vi "MissingIndicator.vi"(8 "error in":errorcluster caption="entrée d'erreur", 11 "MissingIndicator":T1={"missing_values"="nan", "features"="None", "sparse"="None", "error_on_new"=TRUE}) -> (0 "error out":errorcluster caption="sortie d'erreur", 3 "MissingIndicator.lvclass":refnum<class "MissingIndicator.lvclass">)   [LabVIEW 2020]
doc: "Binary indicators for missing values.\n\nNote that this component typically should not be used in a vanilla Pipeline consisting of transformers and a classifier, but rather could be added using a FeatureUnion or ColumnTransformer.\n\nParameters :\n\n- missing_values : number, string, np.nan (default) or None\nThe placeholder for the missing values. All occurrences of missing_values will be imputed. For pandas’ dataframes with nullable integer dtypes with missing values, missing_values should be set to np.nan, since pd.NA will be converted to np.nan.\n\n- features : str, default=None\nWhether the imputer mask should represent all or a subset of features.\n\nIf “missing-only” (default), the imputer mask will only represent features containing missing values during fit time.\n\nIf “all”, the imputer mask will represent all features.\n\n- sparse : boolean or “auto”, default=None\nWhether the imputer mask format should be sparse or dense.\n\nIf “auto” (default), the imputer mask will be of same type as input.\n\nIf True, the imputer mask will be a sparse matrix.\n\nIf False, the imputer mask will be a numpy array.\n\n- error_on_new : boolean, default=None\nIf True (default), transform will raise an error when there are features with missing values in transform that have no missing values in fit. This is applicable only when features=\"missing-only\".\n\n\n\nMethods : \n\n- Fit : Fit the transformer on X.\n\nParameters : X : {array-like, sparse matrix}, shape (n_samples, n_features)\n Input data, where n_samples is the number of samples and n_features is the number of features.\n\n\n- Fit Transform : Generate missing values indicator for X.\n\nParameters : X : {array-like, sparse matrix}, shape (n_samples, n_features)\n The input data to complete.\n\nReturns : Xt {ndarray or sparse matrix}, shape (n_samples, n_features) or (n_samples, n_features_with_missing)\n The missing indicator for input data. The data type of Xt will be boolean.\n\n\n- Transform : Generate missing values indicator for X.\n\nParameters : X : {array-like, sparse matrix}, shape (n_samples, n_features)\n The input data to complete.\n\nReturns : Xt : {ndarray or sparse matrix}, shape (n_samples, n_features) or (n_samples, n_features_with_missing)\n The missing indicator for input data. The data type of Xt will be boolean."
uses:
  MissingIndicator.lvclass
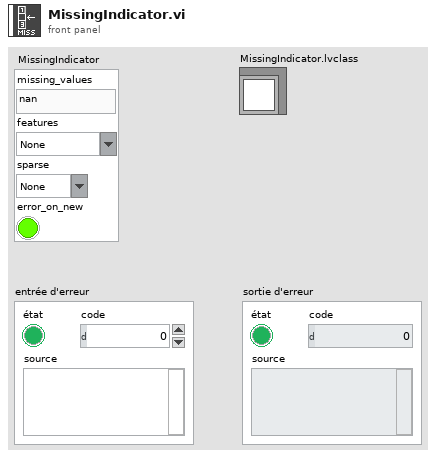
[diagram p1: front panel]
types:
  T1 = cluster{"missing_values":string, "features":string, "sparse":string, "error_on_new":bool}
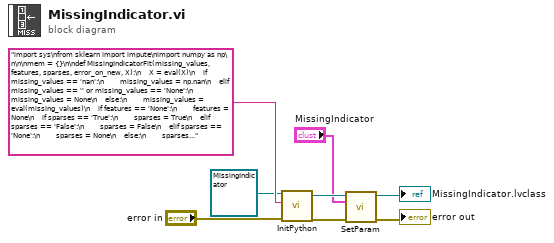
[diagram p0: block diagram]
diagram:
  n1 = call-dynamic "InitPython.vi"("error in (no error)"="error in", "Python Instruction"="import sys\nfrom sklearn import impute\nimport numpy as np\n\n\nmem = {}\n\ndef MissingIndicatorFit(missing_values, features, sparses, error_on_new, X):\n    X = eval(X)\n    if missing_values == 'nan':\n        missing_values = np.nan\n    elif missing_values == '' or missing_values == 'None':\n        missing_values = None\n    else:\n        missing_values = eval(missing_values)\n    if features == 'None':\n        features = None\n    if sparses == 'True':\n        sparses = True\n    elif sparses == 'False':\n        sparses = False\n    elif sparses == 'None':\n        sparses = None\n    else:\n        sparses = 'auto'\n    try:\n        MissingIndicator = impute.MissingIndicator(missing_values, features, sparses, error_on_new).fit(X)\n        mem['FitMissingIndicator'] = MissingIndicator\n        return str('OK')\n    except:\n        erreur = sys.exc_info()\n        typerr = u\"%s\" % (erreur[0])\n        typerr = typerr[typerr.find(\"'\")+1:typerr.rfind(\"'\")]\n        msgerr = u\"%s\" % (erreur[1])\n        message = str('/!\\\\ {0} : {1}'. format(typerr,msgerr))\n        return message \n\ndef MissingIndicatorFitTransform(missing_values, features, sparses, error_on_new, X):\n    X = eval(X)\n    if missing_values == 'nan':\n        missing_values = np.nan\n    elif missing_values == '' or missing_values == 'None':\n        missing_values = None\n    else:\n        missing_values = eval(missing_values)\n    if features == 'None':\n        features = None\n    if sparses == 'True':\n        sparses = True\n    elif sparses == 'False':\n        sparses = False\n    elif sparses == 'None':\n        sparses = None\n    else:\n        sparses = 'auto'\n    try:\n        MissingIndicator = impute.MissingIndicator(missing_values, features, sparses, error_on_new).fit_transform(X)\n        MissingIndicator = MissingIndicator.tolist()\n        return str(MissingIndicator)\n    except:\n        erreur = sys.exc_info()\n        typerr = u\"%s\" % (erreur[0])\n        typerr = typerr[typerr.find(\"'\")+1:typerr.rfind(\"'\")]\n        msgerr = u\"%s\" % (erreur[1])\n        message = str('/!\\\\ {0} : {1}'. format(typerr,msgerr))\n        return message \n    \n\ndef MissingIndicatorTransform(missing_values, features, sparses, error_on_new, X):  \n    X = eval(X)\n    if missing_values == 'nan':\n        missing_values = np.nan\n    elif missing_values == '' or missing_values == 'None':\n        missing_values = None\n    else:\n        missing_values = eval(missing_values)\n    if features == 'None':\n        features = None\n    if sparses == 'True':\n        sparses = True\n    elif sparses == 'False':\n        sparses = False\n    elif sparses == 'None':\n        sparses = None\n    else:\n        sparses = 'auto'\n    try:\n        MissingIndicator = mem['FitMissingIndicator'].transform(X)\n        MissingIndicator = MissingIndicator.tolist()\n        return str(MissingIndicator)\n    except:\n        erreur = sys.exc_info()\n        typerr = u\"%s\" % (erreur[0])\n        typerr = typerr[typerr.find(\"'\")+1:typerr.rfind(\"'\")]\n        msgerr = u\"%s\" % (erreur[1])\n        message = str('/!\\\\ {0} : {1}'. format(typerr,msgerr))\n        return message", "Scikit-learn en entrée"=refnum<class "MissingIndicator.lvclass"> refnum ("MissingIndicator.lvclass")) -> ("error out"=w4:errorcluster, "Scikit-learn en sortie"=w5:refnum<class "MissingIndicator.lvclass">)  [unwired: 7 in]
  n2 = call-dynamic "SetParam.vi"("error in (no error)"=w4, "MissingIndicator"="MissingIndicator", "MissingIndicator.lvclass"=w5) -> ("error out"=→"error out":errorcluster, "MissingIndicator.lvclass"=→"MissingIndicator.lvclass":refnum<class "MissingIndicator.lvclass">)  [unwired: 7 in]
